vi "MeasureRMS.vi"(10 "Input Parameters":T1) -> (1 "Waveform Graph":dynamicdata(graph), 2 "RMS Output":dbl format="%0.2f")   [LabVIEW 2014]
uses:
  <vilib>/Analysis/NI_AALPro.lvlib
panel:
  out "error out":errorcluster
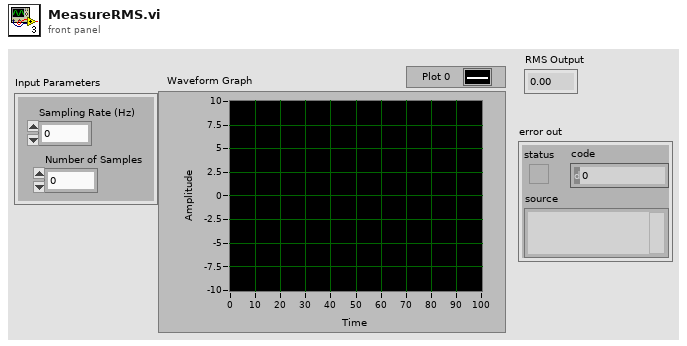
[diagram p1: front panel]
types:
  T1 = cluster{"Sampling Rate (Hz)":dbl, "Number of Samples":dbl}
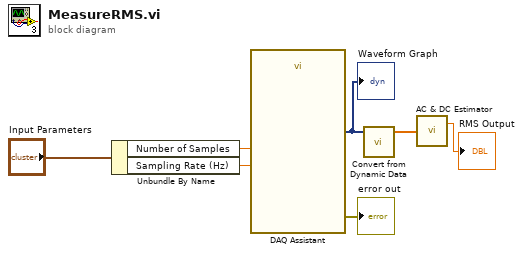
[diagram p0: block diagram]
diagram:
  n1 = Unbundle By Name("Input Parameters") -> ("Number of Samples"=w1:dbl, "Sampling Rate (Hz)"=w2:dbl)
  n2 = call "DAQ Assistant"("rate"=w2, "number of samples"=w1) -> ("data"=w7:dynamicdata, "error out"=→"error out":errorcluster)  [unwired: 15 in, 1 out]
  "Waveform Graph" <- w7
  n3 = call "Convert from Dynamic Data"("Dynamic Data Type"=w7) -> ("Array"=w6:dbl[])  [unwired: 3 in]
  n4 = call <vilib>:"AC & DC Estimator.vi"("Signal (V)"=w6) -> ("AC estimate (Vrms)"=→"RMS Output":dbl)  [unwired: 1 out]
